vi "Limelight Set Mode Vision Processor or Camera.vi"(9 "Limelight Mode\n0 = Vision Processor\n1 = Camara":dbl format="%#_13g", 11 "Cam Mode":bool) -> ()   [LabVIEW 2020]
uses:
  <vilib>/Rock Robotics/Network Tables/NT Write Number.vi
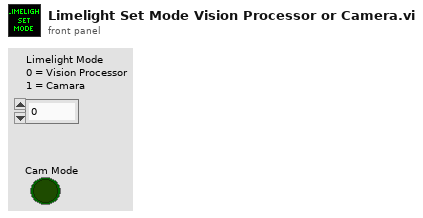
[diagram p1: front panel]
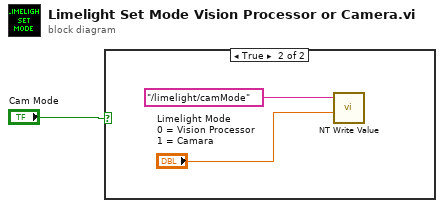
[diagram p0: block diagram]
diagram:
  n1 = case shown="True" "Cam Mode" {
    frame False {
    }
    frame True {
      n2 = call-poly <vilib>:"NT Write Value.vi"("Numeric"="Limelight Mode\n0 = Vision Processor\n1 = Camara", "Name"="/limelight/camMode") -> ()  [unwired: 9 in, 1 out]
    }
  }
